vi "Load XML with Parser API.vi"() -> ()   [LabVIEW 2023]
doc: "This example loads test configuration data from an XML file, and checks to see if it is valid against a specific schema. Select whether you want to load the valid or invalid file and run the VI to see the results."
uses:
  support/Helper - Test Settings.ctl
  <vilib>/xml/Load XML File.vi
  <vilib>/xml/Close Reference(Node).vi
  <vilib>/xml/Close Reference(NdList).vi
  <resource>/objmgr/DOMUserDefRef.rc
  <vilib>/xml/NI_XML.lvlib
panel:
  in  "Schema Type":u16(ring) items=["Valid", "Invalid"]
  out "Test Configuration":T1[](array[typedef])
  out "Parse Errors":string
  out "XML File Path":path
  # "Overview: Demonstrates the use of the XML Parser VIs and functions to load an XML file, validate it against a known schema, and parse its contents.\nInstructions:\n1. Specify a Schema Type of 'Valid' and run the VI. The contents of the XML file will be displayed in the Test Configuration indicator.\n2. Specify a Schema Type of 'Invalid' and run the VI. Since the invalid XML does not validate properly against its schema, several Parse Errors will be displayed, and error -2628 will occur."
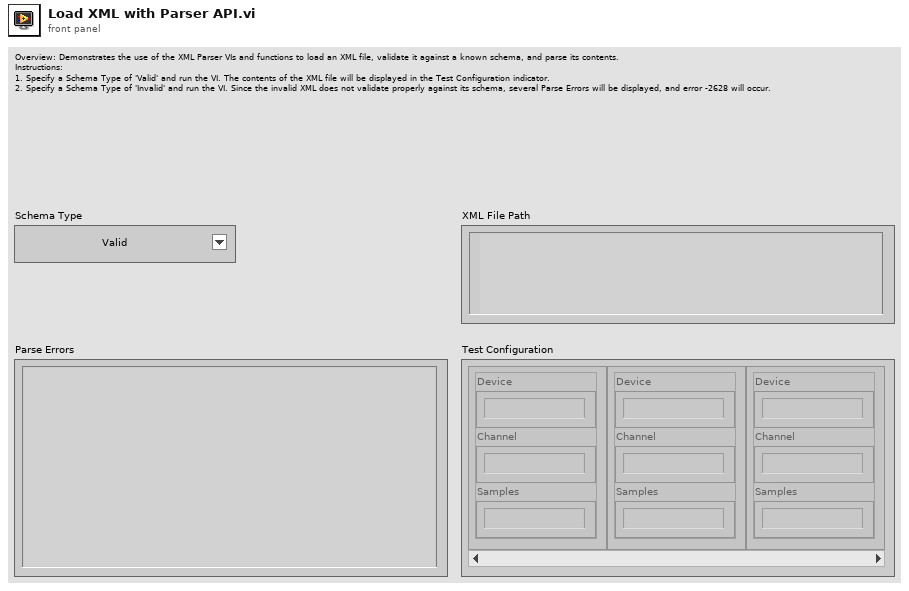
[diagram p1: front panel]
types:
  T1 = typedef "Helper - Test Settings.ctl" = cluster{"Device":string, "Channel":string, "Samples":string}
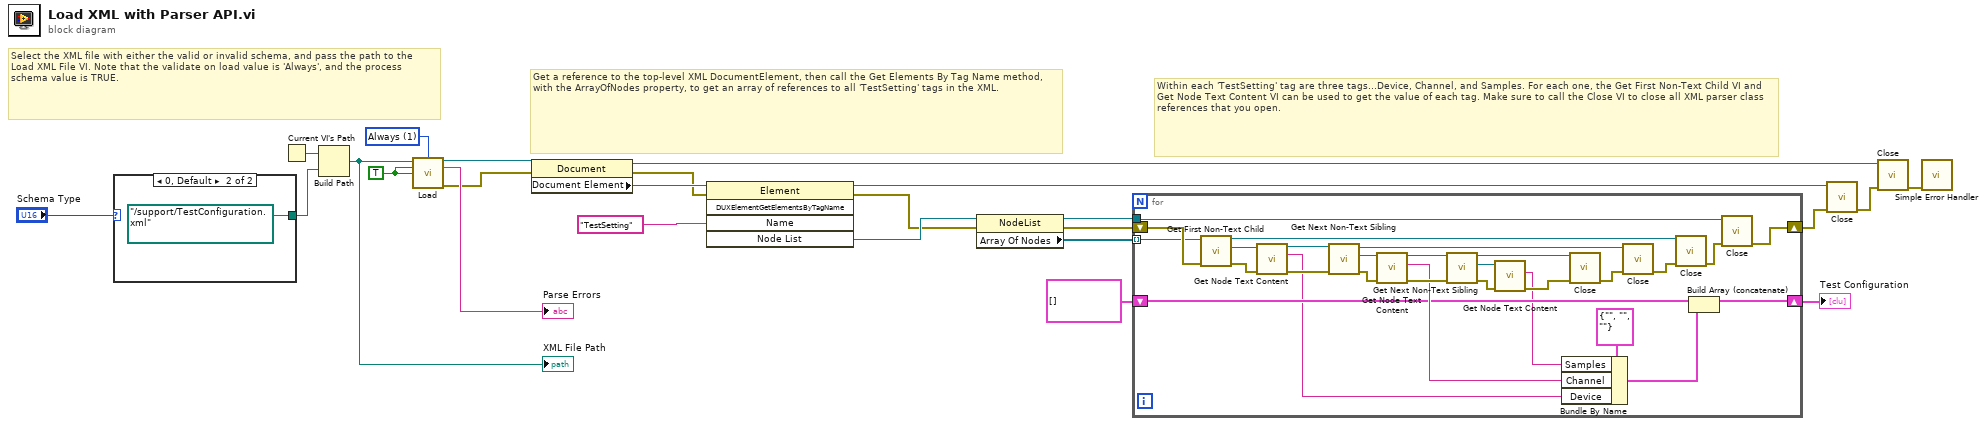
[diagram p0: block diagram]
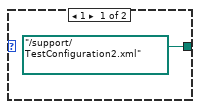
[diagram p2: hidden frame]
diagram:
  w24 = 1 items=["Never", "Always", "Auto"] ("Validate On Load")
  w1 = TRUE ("Do Namespaces")
  # "Within each 'TestSetting' tag are three tags...Device, Channel, and Samples. For each one, the Get First Non-Text Child VI and Get Node Text Content VI can be used to get the value of each tag. Make sure to call the Close VI to close all XML parser class references that you open."
  # "Get a reference to the top-level XML DocumentElement, then call the Get Elements By Tag Name method, with the ArrayOfNodes property, to get an array of references to all 'TestSetting' tags in the XML."
  # "Select the XML file with either the valid or invalid schema, and pass the path to the Load XML File VI. Note that the validate on load value is 'Always', and the process schema value is TRUE."
  n1 = case shown="0, Default" "Schema Type" {
    tunnel: [path "../support/TestConfiguration2.xml" path "../support/TestConfiguration.xml"] -> w5
    frame 1 {
    }
    frame 0, Default {
    }
  }
  n2 = Current VI's Path() -> (path=w2:path)
  n3 = Build Path(base path=w2, name or relative path=w5) -> (appended path=w6:path)
  "XML File Path" <- w6
  n4 = call-poly <vilib>:"Load.vi"("path to XML document"=w6, "validate on load (Auto)"=w24, "process namespaces (False)"=w1, "process schema (False)"=w1) -> ("DOM document out"=w8:refnum<k20>, "parse errors"=→"Parse Errors":string, "error out"=w7:errorcluster)  [unwired: 3 in, 6 out]
  n5 = property class="Document"(reference=w8, error in=w7) -> (reference out=w9:refnum<k20>, error out=w20:errorcluster, "Document Element"=w21:refnum<k20>)
  n6 = invoke class="Element" method="DUXElementGetElementsByTagName"(reference=w21, error in=w20, "Name"="TestSetting" ("Node Name")) -> (reference out=w11:refnum<k20>, error out=w18:errorcluster, "Node List"=w19:refnum<k20>)  [unwired: 2 in, 2 out]
  n7 = property class="NodeList"(reference=w19, error in=w18) -> (reference out=w17:refnum<k20>, error out=w15:errorcluster, "Array Of Nodes"=w13:refnum<k20>[])
  n8 = for {
    tunnel: w13 -> [w30] mode=indexing
    tunnel: w17 -> [w38]
    shift-right: [w33] -> w14
    shift-left: T1[] [] -> [w35]
    shift-right: [w37] -> w12
    shift-left: w15 -> [w32]
    n9 = call <vilib>:"Get First Non-Text Child.vi"("error in (no error)"=w32, "node in"=w30) -> ("error out"=w53:errorcluster, "child node"=w54:refnum<k20>, "node out"=w46:refnum<k20>)  [unwired: 7 out]
    n10 = call <vilib>:"Get Node Text Content.vi"("error in (no error)"=w53, "node in"=w54) -> ("error out"=w49:errorcluster, "node text"=w27:string, "node out"=w50:refnum<k20>)  [unwired: 7 out]
    n11 = call <vilib>:"Get Next Non-Text Sibling.vi"("error in (no error)"=w49, "node in"=w50) -> ("error out"=w52:errorcluster, "sibling node"=w51:refnum<k20>, "node out"=w48:refnum<k20>)  [unwired: 7 out]
    n12 = call <vilib>:"Get Node Text Content.vi"("error in (no error)"=w52, "node in"=w51) -> ("error out"=w42:errorcluster, "node text"=w36:string, "node out"=w44:refnum<k20>)  [unwired: 7 out]
    n13 = call <vilib>:"Get Next Non-Text Sibling.vi"("error in (no error)"=w42, "node in"=w44) -> ("error out"=w41:errorcluster, "sibling node"=w40:refnum<k20>, "node out"=w43:refnum<k20>)  [unwired: 7 out]
    n14 = call <vilib>:"Get Node Text Content.vi"("error in (no error)"=w41, "node in"=w40) -> ("error out"=w39:errorcluster, "node text"=w28:string)  [unwired: 8 out]
    n15 = Bundle By Name(cluster=T1 {"Device"="", "Channel"="", "Samples"=""} ("Test Settings"), "Samples"=w28, "Channel"=w36, "Device"=w27) -> (w34:T1)
    n16 = call-poly <vilib>:"Close.vi"("error in (no error)"=w39, "node"=w43) -> ("error out"=w47:errorcluster)  [unwired: 7 out]
    n17 = call-poly <vilib>:"Close.vi"("error in (no error)"=w47, "node"=w48) -> ("error out"=w45:errorcluster)  [unwired: 7 out]
    n18 = call-poly <vilib>:"Close.vi"("error in (no error)"=w45, "node"=w46) -> ("error out"=w31:errorcluster)  [unwired: 7 out]
    n19 = Build Array (concatenate)(w35, w34) -> (w33:T1[])
    n20 = call-poly <vilib>:"Close.vi"("error in (no error)"=w31, "node list"=w38) -> ("error out"=w37:errorcluster)  [unwired: 7 out]
  }
  "Test Configuration" <- w14
  n21 = call-poly <vilib>:"Close.vi"("error in (no error)"=w12, "node"=w11) -> ("error out"=w10:errorcluster)  [unwired: 7 out]
  n22 = call-poly <vilib>:"Close.vi"("error in (no error)"=w10, "node"=w9) -> ("error out"=w3:errorcluster)  [unwired: 7 out]
  n23 = call <vilib>:"Simple Error Handler.vi"("error in (no error)"=w3) -> ()  [unwired: 4 in, 5 out]
